vi "Word_Print.vi"(0 "Word._Application":refnum<k7>, 1 "Word._Document":refnum<k7>, 7 "printer name (default)":string, 9 "number of copies (1)":i32, 11 "error in (no error)":errorcluster) -> (15 "error out":errorcluster)   [LabVIEW 2010, in "NI_ReportGenerationToolkit.lvlib"]
uses:
  <vilib>/addons/_office/NI_ReportGenerationToolkit.lvlib
  <vilib>/Utility/NIReport.llb/NI_ReportGenerationCore.lvlib
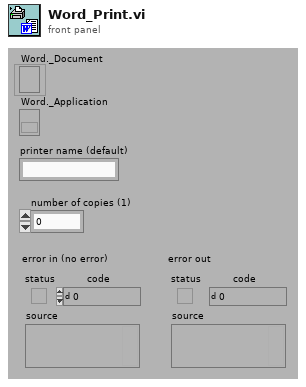
[diagram p1: front panel]
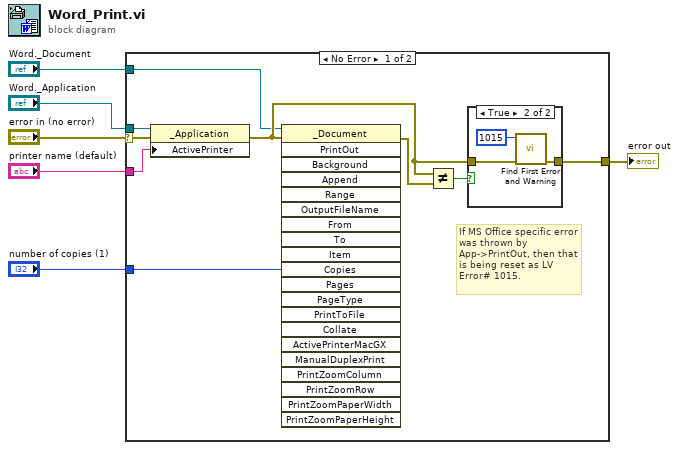
[diagram p0: block diagram]
diagram:
  n1 = case shown="No Error" "error in (no error)" {
    selector: "error in (no error)" -> [w9 w20]
    tunnel: "Word._Application" -> [w15 _]
    tunnel: [w14 w20] -> w5
    tunnel: "number of copies (1)" -> [w7 _]
    tunnel: "printer name (default)" -> [w10 _]
    tunnel: "Word._Document" -> [w8 _]
    frame No Error {
      # "If MS Office specific error was thrown by App->PrintOut, then that is being reset as LV Error# 1015."
      n2 = property class="_Application"(reference=w15, error in=w9, "ActivePrinter"=w10) -> (error out=w11:errorcluster)  [unwired: 1 out]
      n3 = invoke class="_Document" method="PrintOut"(reference=w8, error in=w11, "Copies"=w7) -> (error out=w13:errorcluster)  [unwired: 18 in, 20 out]
      n4 = Not Equal?(x=w11, y=w13) -> (x != y?=w12:bool)
      n5 = case shown="True" w12 {
        tunnel: w11 -> [w16 w18]
        tunnel: [w16 w17] -> w14
        frame False {
        }
        frame True {
          n6 = call <vilib>:"Find First Error and Warning.vi"("error in (no error)"=w18, "error code"=1015) -> ("error out"=w17:errorcluster)  [unwired: 5 out]
        }
      }
    }
    frame Error {
    }
  }
  "error out" <- w5
